vi "Process.vi"(0 "reference in":refnum<class "Script.lvclass">, 5 "error in":errorcluster) -> (14 "reference out":refnum<class "Script.lvclass">, 19 "error out":errorcluster)   [LabVIEW 2023, in "Script.lvclass"]
uses:
  Script.lvclass
  Script.lvclass/Script.ctl
  <vilib>/Utility/SystemLogging/NI_SystemLogging.lvlib
panel:
  out "error info":errorcluster
  out "Last Command":string
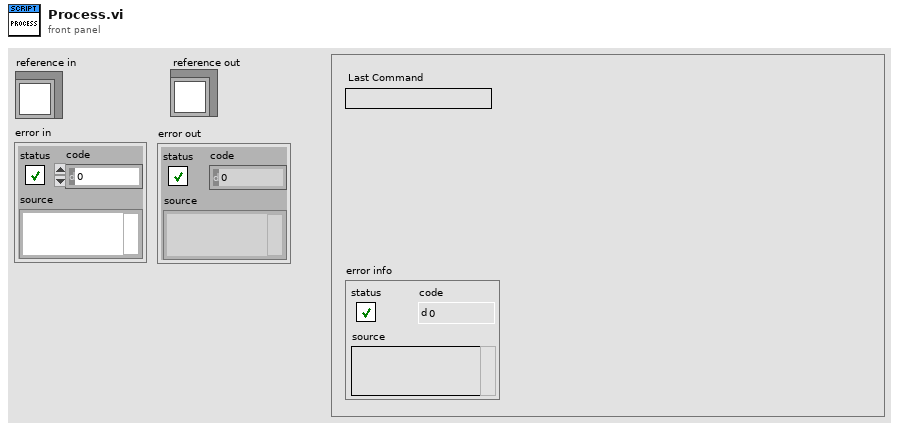
[diagram p1: front panel]
types:
  T1 = cluster{"Core":cluster{"Timeout":i32, "Events":cluster{"EventsToProcess":refnum<event-registration>}, "EventFromProcess":refnum<user-event>, "ProcessSyncQueue":refnum<queue>, "QueueFromProcess":refnum<queue>, "Command":string, "Data":variant}, "Process ID":i32, "Script Prefix":string, "Log File":string, "Full Command":string, "Script Name":string, "Console Listbox":refnum<vi>}
  T2 = enum32{"Invalid", "Standard", "Closed", "Hidden", "Minimized", "Maximized"}
  T3 = cluster{"EventsToProcess":refnum<event-registration>}
  T4 = typedef "Script.lvclass/ObjectAttributes.ctl" = cluster{"Update Rate (ms)":i32, "Console Listbox":refnum<vi>, "Full Command":string, "Script Name":string, "Log File":string, "IP Address":string}
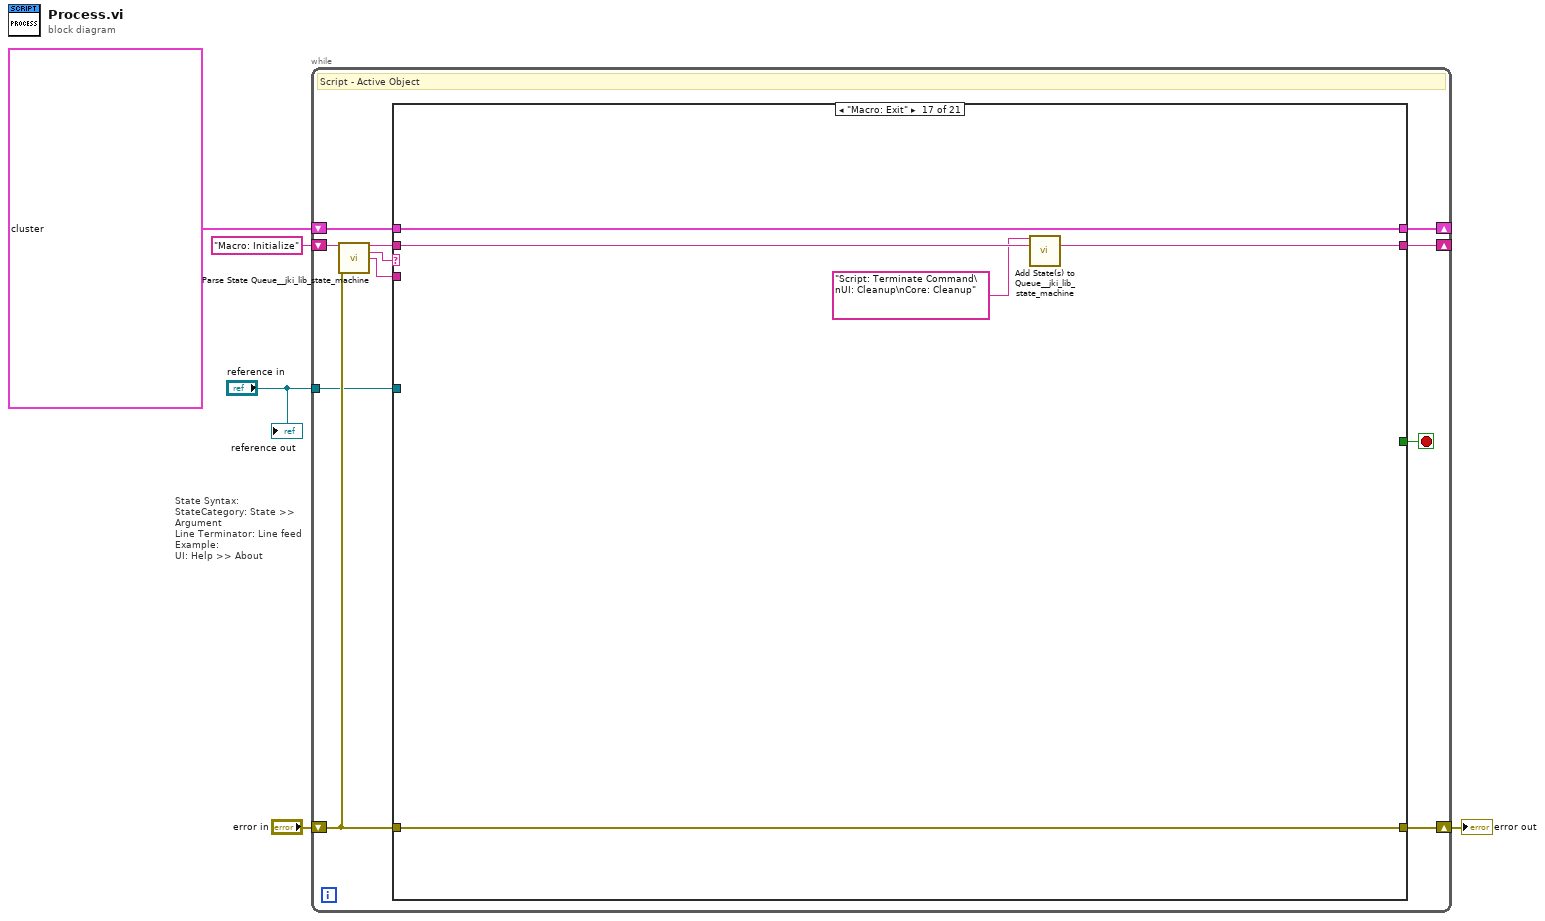
[diagram p0: block diagram]
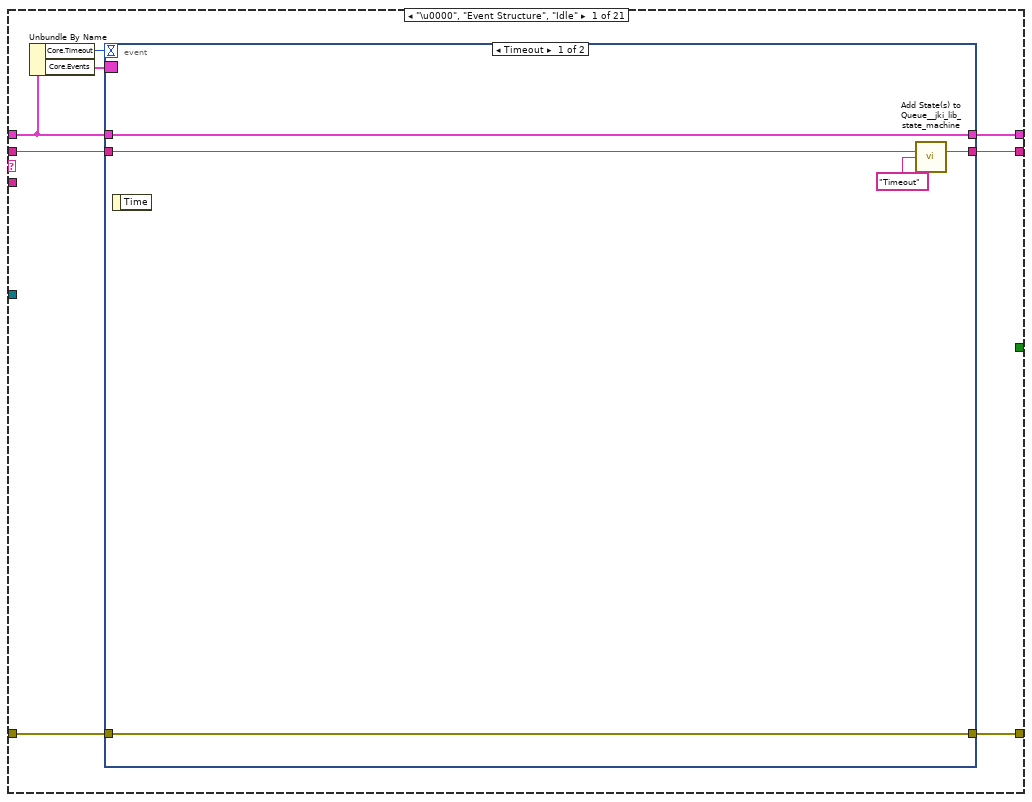
[diagram p2: hidden frame]
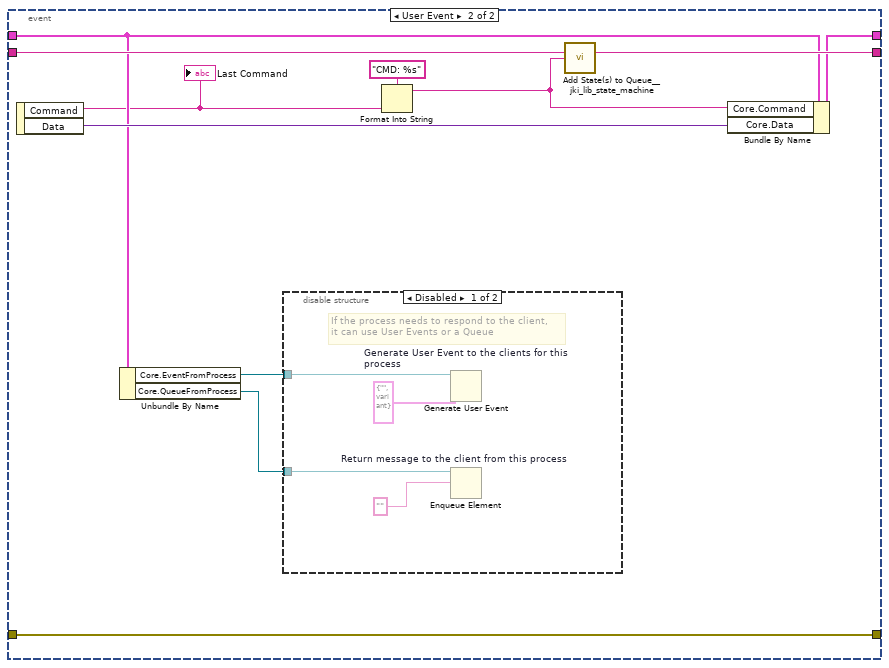
[diagram p3: hidden frame]
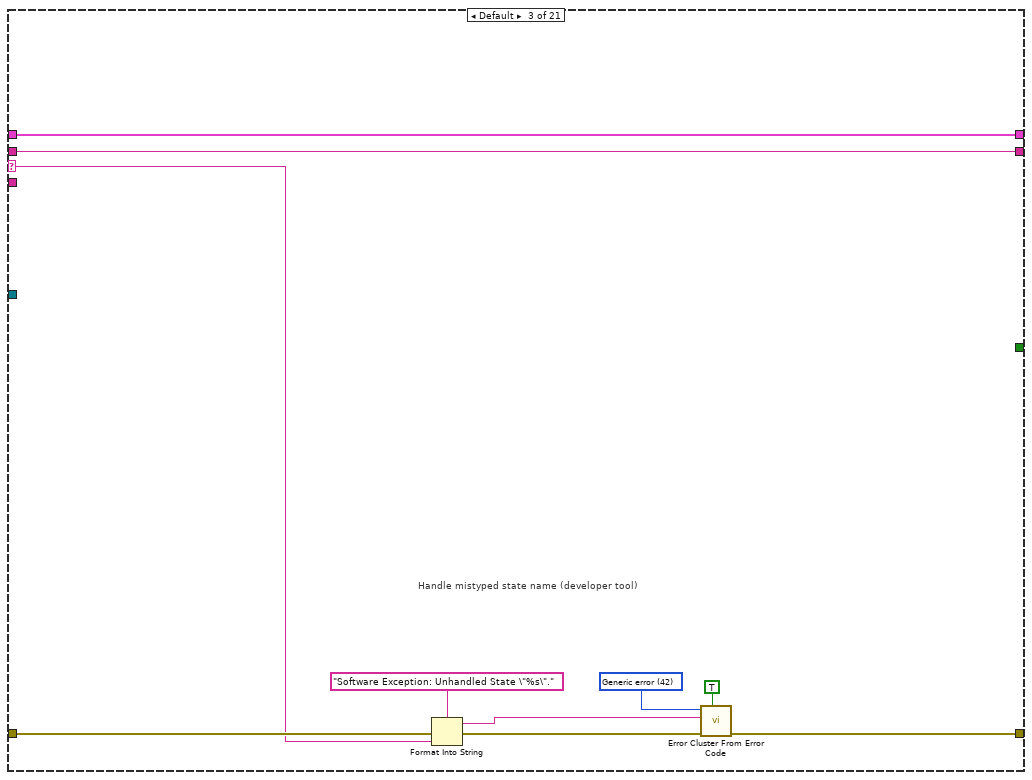
[diagram p6: hidden frame]
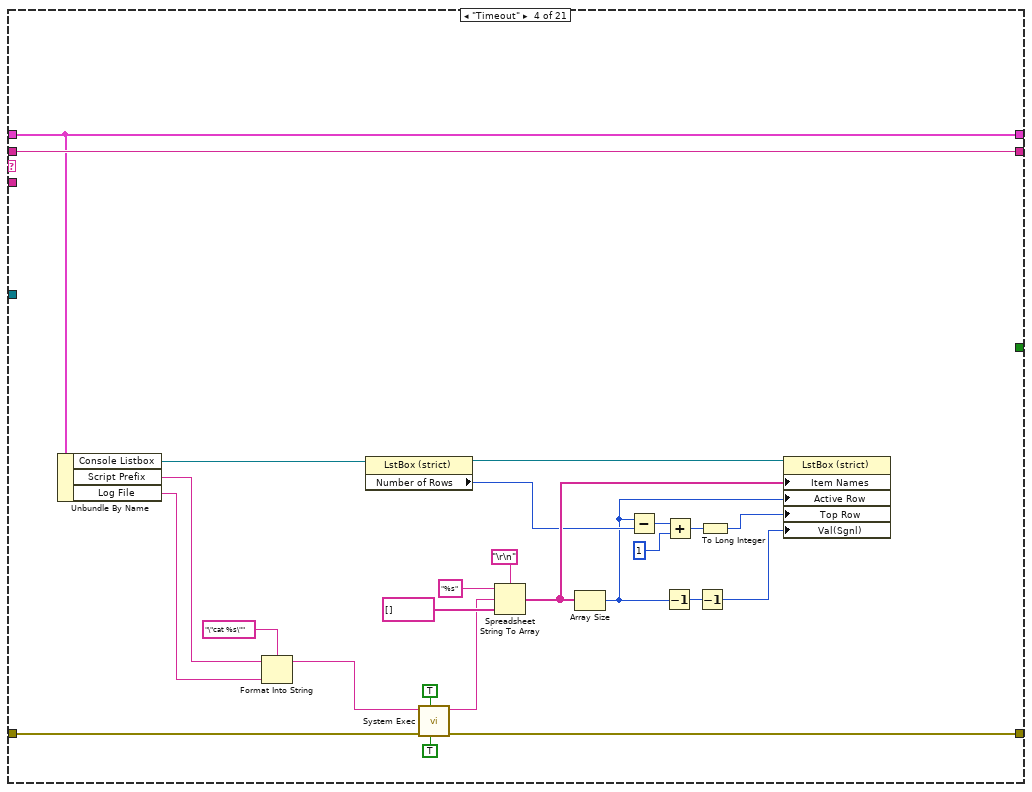
[diagram p7: hidden frame]
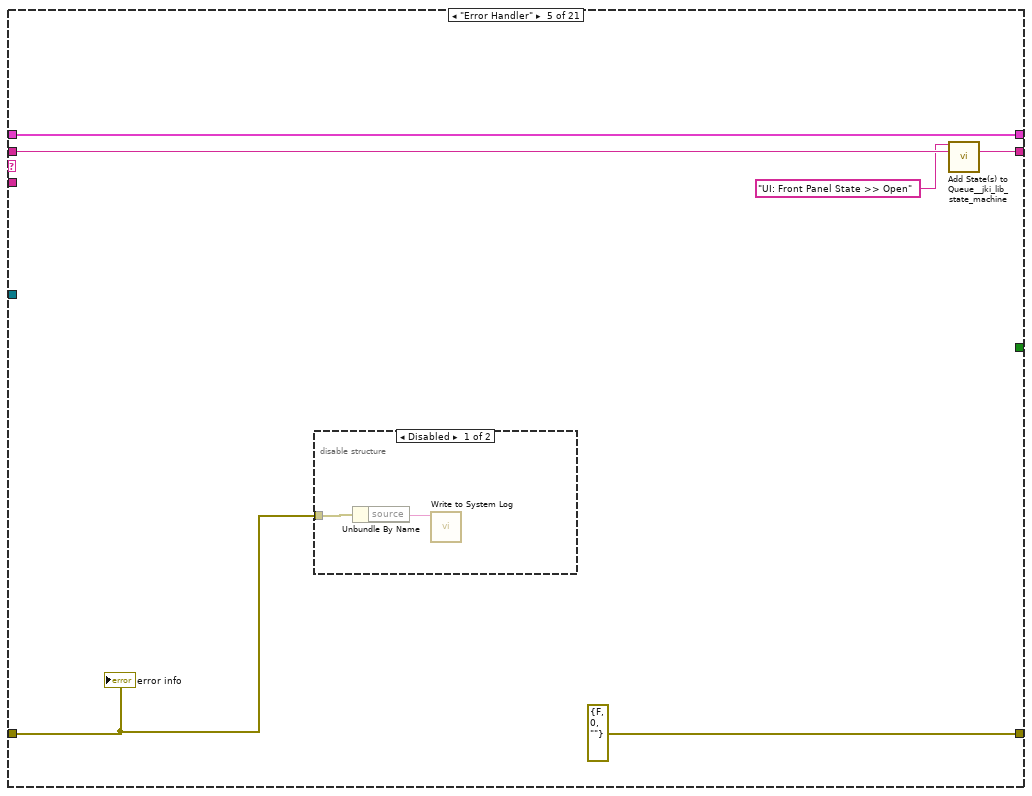
[diagram p8: hidden frame]
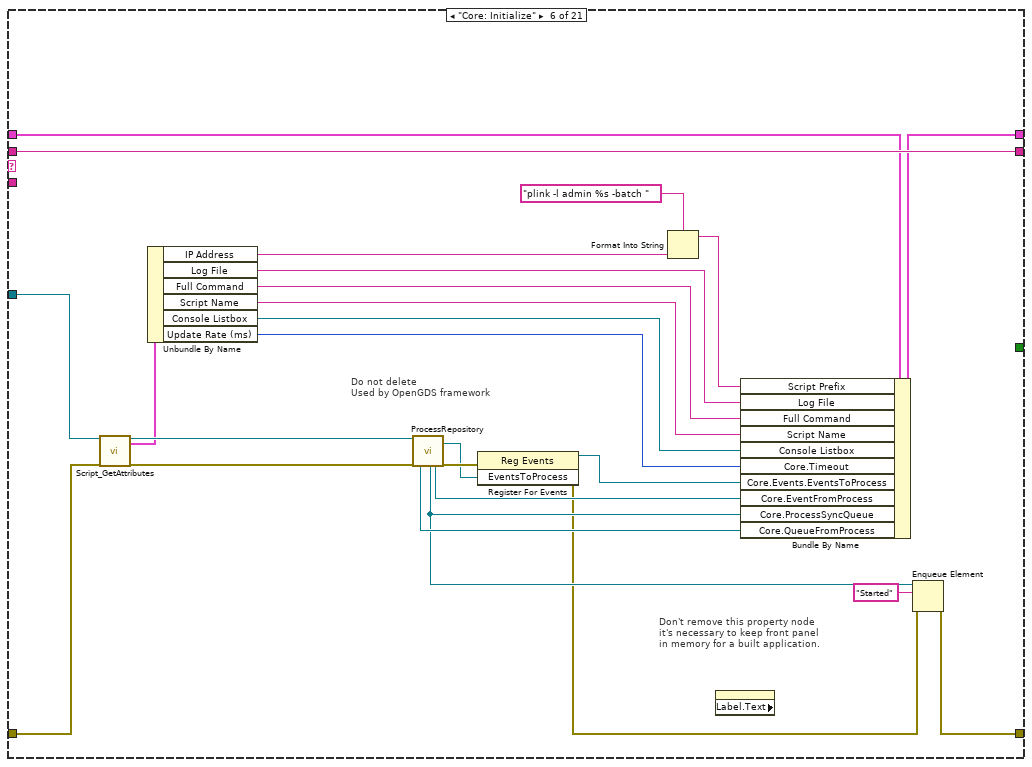
[diagram p10: hidden frame]
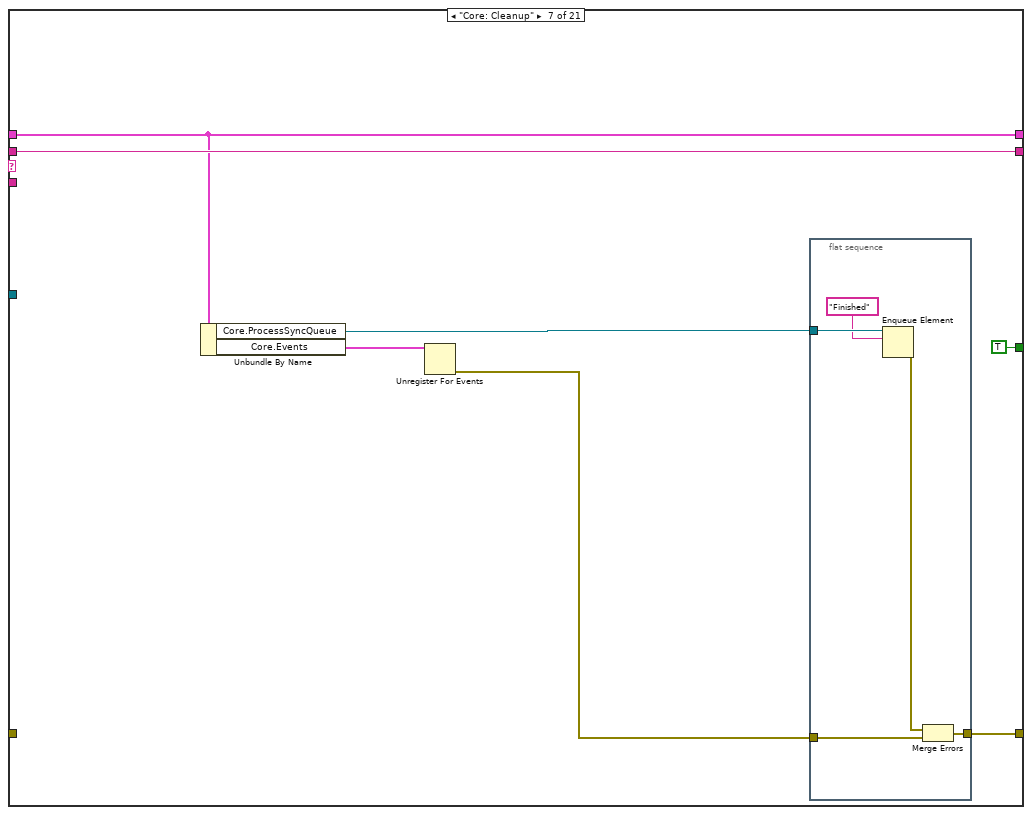
[diagram p11: hidden frame]
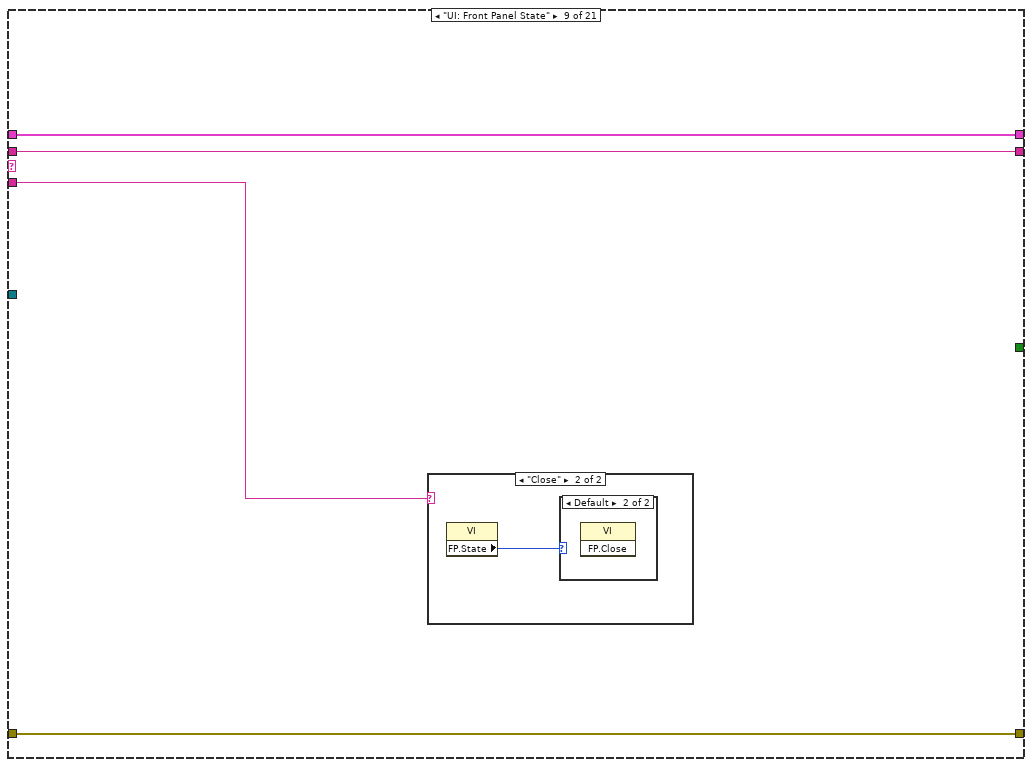
[diagram p13: hidden frame]
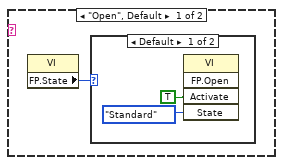
[diagram p14: hidden frame]
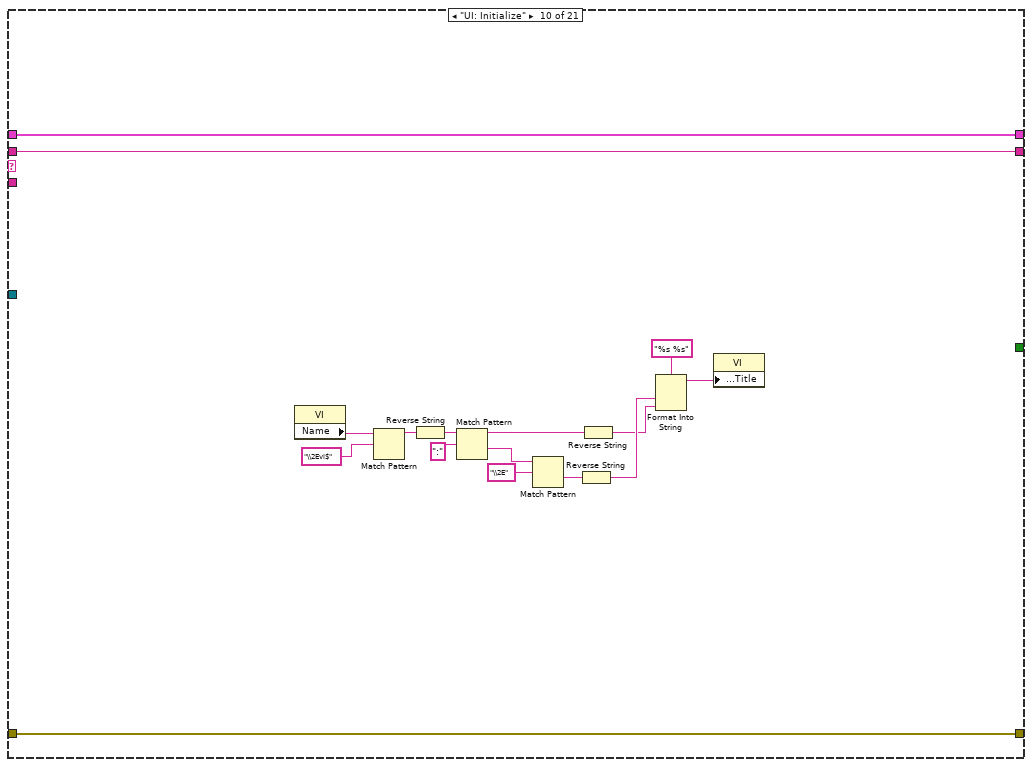
[diagram p17: hidden frame]
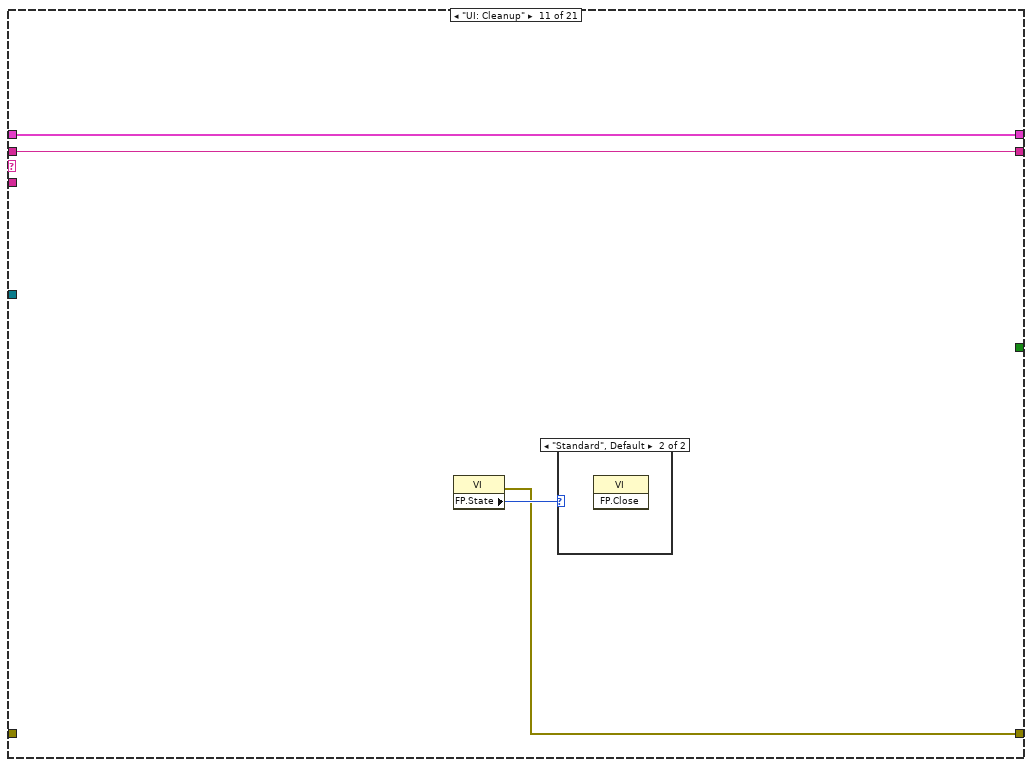
[diagram p18: hidden frame]
diagram:
  # "State Syntax:\nStateCategory: State >> Argument\nLine Terminator: Line feed\nExample:\nUI: Help >> About"
  n1 = while {
    shift-right: [w15] -> w4
    shift-left: "error in" -> [w16]
    shift-right: [w8] -> _
    shift-left: "Macro: Initialize" ("States Out") -> [w11]
    shift-right: [w14] -> _
    shift-left: T1 {"Core"={"Timeout"=-1, "Events"={"EventsToProcess"=refnum}, "EventFromProcess"=refnum, "ProcessSyncQueue"=refnum, "QueueFromProcess"=refnum, "Command"="", "Data"=variant}, "Process ID"=0, "Script Prefix"="", "Log File"="", "Full Command"="", "Script Name"="", "Console Listbox"=refnum} ("LocalVariables") -> [w13]
    tunnel: "reference in" -> [w6]
    stop <- w7 stop-if-true
    # "Script - Active Object"
    n2 = call <vilib>:"Parse State Queue__jki_lib_state_machine.vi"("State Queue"=w11, "Error In (no error)"=w16) -> ("Remaining States"=w10:string, "Current State"=w12:string, "Arguments"=w9:string)  [unwired: 11 in]
    n3 = case shown="\"Macro: Exit\"" w12 {
      selector: w12 -> [_ _ w48 _ _ _ _ _ _ _ _ _ _ _ _ _ _ _ _ _ _]
      tunnel: w16 -> [w18 w47 w50 w63 w84 w101 _ w130 w131 w154 _ w161 w164 w171 w172 w178 w183 w185 w193 w202 w219]
      tunnel: [w19 w47 w49 w62 errorcluster {"status"=FALSE, "code"=0, "source"=""} ("error constant") w115 w118 w130 w131 w154 w155 w161 w164 w171 w172 w178 w183 w185 w192 w201 w217] -> w15
      tunnel: [w24 w46 w57 w61 w88 w113 w119 w129 w133 w146 w156 w160 w163 w170 w173 w179 w184 w186 w190 w203 w216] -> w14
      tunnel: w13 -> [w20 w46 w57 w61 w88 w112 w119 w129 w133 w146 w156 w160 w163 w170 w173 w179 w184 w186 w191 w203 w216]
      tunnel: w10 -> [w22 w45 w56 w82 w87 w114 w122 w128 w134 w153 w158 w159 _ w169 w174 w177 w182 w187 w200 w209 w221]
      tunnel: w9 -> [_ _ _ _ _ _ _ _ w132 _ _ _ _ w166 _ _ _ _ _ _ _]
      tunnel: [w21 w45 w56 w82 w86 w114 w122 w128 w134 w153 w158 w159 "Macro: Exit" ("State(s) at Back (\"\")") w168 w174 w176 w181 w187 w200 w209 w221] -> w8
      tunnel: [_ _ _ _ _ _ TRUE _ _ _ _ _ _ _ _ _ _ _ _ _ _] -> w7
      tunnel: w6 -> [_ _ _ _ _ w103 _ _ _ _ _ _ _ _ _ _ _ _ _ _ _]
      frame "\u0000", "Event Structure", "Idle" {
        n4 = Unbundle By Name(w20) -> ("Core.Timeout"=w17:i32, "Core.Events"=w23:T3)
        n5 = event shown="[0] Timeout" {
          selector: w23 -> [_ _]
          dyn-events: _ -> [_ _]
          timeout: w17 -> [_ _]
          tunnel: w20 -> [w29 w33]
          tunnel: [w29 w38] -> w24
          tunnel: [w27 w40] -> w21
          tunnel: w22 -> [w28 w39]
          tunnel: [w25 w34] -> w19
          tunnel: w18 -> [w25 w34]
          event Timeout {
            n6 = event-data() -> ()  [unwired: 1 in, 1 out]
            n7 = call <vilib>:"Add State(s) to Queue__jki_lib_state_machine.vi"("State(s) in (\"\")"=w28, "State(s) at Back (\"\")"="Timeout" ("State(s) at Back (\"\")")) -> ("States Out"=w27:string)  [unwired: 13 in]
          }
          event User Event {
            n8 = event-data() -> ("Command"=w31:string, "Data"=w37:variant)  [unwired: 1 in]
            "Last Command" <- w31
            n9 = Unbundle By Name(w33) -> ("Core.EventFromProcess"=w36:refnum<user-event>, "Core.QueueFromProcess"=w35:refnum<queue>)
            n10 = disable-structure shown="Disabled" {
              disable-tunnel: w36 -> [w44 _]
              disable-tunnel: w35 -> [w43 _]
              frame Disabled {
                # "If the process needs to respond to the client,\nit can use User Events or a Queue"
                n11 = Generate User Event "Generate User Event to the clients for this process"(user event=w44, event data cluster=cluster{"Command":string, "Data":variant} {"Command"="", "Data"=variant} ("event data")) -> ()  [unwired: 2 in, 2 out]
                n12 = Enqueue Element "Return message to the client from this process"(queue=w43, element="") -> ()  [unwired: 2 in, 3 out]
              }
              frame Enabled {
              }
            }
            n13 = Format Into String(format string="CMD: %s", w31) -> (resulting string=w30:string)  [unwired: 2 in, 1 out]
            n14 = call <vilib>:"Add State(s) to Queue__jki_lib_state_machine.vi"("State(s) in (\"\")"=w39, "State(s) at Back (\"\")"=w30) -> ("States Out"=w40:string)  [unwired: 13 in]
            n15 = Bundle By Name(cluster=w33, "Core.Command"=w30, "Core.Data"=w37) -> (w38:T1)
          }
        }
      }
      frame "---------- Core ----------" {
      }
      frame Default {
        w54 = 42 items=["No error", "Argument error", "Memory is full", "Out of zone", "End of file", "File already open", "Generic file I/O error", "File not found", "File permission error", "Disk is full", "Duplicate path", "Too many files open", "System feature not enabled", "Resource file not found", "Cannot add resource", "Resource not found", "Image not found", "Image memory error", "Pen does not exist", "Config type invalid", "Config token not found", "Config parse error", "Config memory error", "Bad external code format", "Bad external code offset", "External code not present", "Null window", "Destroy window error", "Null menu", "Print aborted", "Bad print record", "Print driver error", "Windows error during printing", "Memory error during printing", "Print dialog error", "Generic print error", "Invalid device refnum", "Device not found", "Device parameter error", "Device unit error", "Cannot open device", "Device call aborted", "Generic error", "Cancelled by user", "Object ID too low", "Object ID too high", "Object not in heap", "Unknown heap", "Unknown object (invalid DefProc)", "Unknown object (DefProc not in table)", "Message out of range", "Invalid (null) method", "Unknown message", "Manager call not supported", "Bad address", "Network operation in progress", "Network operation timed out", "Connection is busy", "Network attribute not supported", "Network error", "Address in use", "System out of memory", "Connection aborted", "Connection refused", "Not connected", "Already connected", "Connection closed", "Initialization error (interapplication manager)", "Bad occurrence", "Wait on unbound occurrence handler", "Occurrence queue overflow", "Datalog type conflict", "Unused", "Unrecognized type (interapplication manager)", "Memory corrupt", "Failed to make temporary DLL", "Old CIN version", "Drag socket not found", "Failed to load drop-object", "Failed to register OLE object", "Failed to release OLE object", "Format specifier type mismatch", "Unknown format specifier", "Too few format specifiers", "Too many format specifiers", "Scan failed", "Newer CIN version", "Error converting to variant", "Runtime menu error", "Password tampered", "Variant attribute not found", "Incompatible variant data type", "Event data is not available", "Event Store is not present", "Occurrence is not found", "Event Queue is not created", "Event info is not available", "Refnum passed is NULL", "Error retrieving Class GUID", "Error retrieving CoClass GUID", "Error retrieving TypeLib GUID.", "Bad built application magic bytes.", "Specific driver is different from the specific driver associated with the Logical Name.", "There is no session opened to the class driver.", "Max Error", "MAX - Error with config objects", "MAX - Error loading configuration", "MAX - Group not supported"]
        # "Handle mistyped state name (developer tool)"
        n16 = Format Into String(format string="Software Exception: Unhandled State \"%s\"." ("message"), error in=w50, w48) -> (resulting string=w53:string, error out=w52:errorcluster)  [unwired: 1 in]
        n17 = call <vilib>:"Error Cluster From Error Code.vi"("show call chain? (False)"=TRUE, "error in (no error)"=w52, "error message (\"\")"=w53, "error code (0)"=w54) -> ("error out"=w49:errorcluster)  [unwired: 5 in]
      }
      frame "Timeout" {
        n18 = Unbundle By Name(w61) -> ("Console Listbox"=w60:refnum<vi>, "Script Prefix"=w58:string, "Log File"=w59:string)
        n19 = Format Into String(format string="\"cat %s\"", initial string=w58, w59) -> (resulting string=w78:string)  [unwired: 1 in, 1 out]
        n20 = property class="LstBox (strict)"(reference=w60) -> (reference out=w73:refnum<vi>, "Number of Rows"=w67:u32)  [unwired: 1 in, 1 out]
        n21 = call <vilib>:"System Exec.vi"("run minimized? (F)"=TRUE, "wait until completion? (T)"=TRUE, "error in (no error)"=w63, "command line"=w78) -> ("error out"=w62:errorcluster, "standard output"=w76:string)  [unwired: 4 in, 2 out]
        n22 = Spreadsheet String To Array(delimiter (Tab)="\r\n", format string="%s", spreadsheet string=w76, array type (2D Dbl)=string[] []) -> (array=w68:string[])
        n23 = Array Size(array=w68) -> (size(s)=w65:i32)
        n24 = Subtract(x=w65, y=w67) -> (x-y=w72:u32)
        n25 = Decrement(x=w65) -> (x-1=w64:i32)
        n26 = Add(x=w72, y=u32 1) -> (x+y=w70:u32)
        n27 = Decrement(x=w64) -> (x-1=w66:i32)
        n28 = To Long Integer(number=w70) -> (32bit integer=w69:i32)
        n29 = property class="LstBox (strict)"(reference=w73, "Item Names"=w68, "Active Row"=w65, "Top Row"=w69, "Val(Sgnl)"=w66) -> ()  [unwired: 1 in, 2 out]
      }
      frame "Error Handler" {
        n30 = disable-structure shown="Disabled" {
          disable-tunnel: w84 -> [w90 _]
          frame Disabled {
            n31 = Unbundle By Name(w90) -> ("source"=w89:string)
            n32 = call <vilib>:"Write to System Log.vi"("message"=w89) -> ()  [unwired: 10 in, 1 out]
          }
          frame Enabled {
          }
        }
        n33 = call <vilib>:"Add State(s) to Queue__jki_lib_state_machine.vi"("State(s) in Front (\"\")"="UI: Front Panel State >> Open" ("State(s) at Back (\"\")"), "State(s) in (\"\")"=w87) -> ("States Out"=w86:string)  [unwired: 13 in]
        "error info" <- w84
      }
      frame "Core: Initialize" {
        # "Do not delete\nUsed by OpenGDS framework"
        # "Don't remove this property node\nit's necessary to keep front panel\nin memory for a built application."
        # "Template created by VI Technologies"
        n34 = call "Script_GetAttributes.vi"("reference in"=w103, "Error In"=w101) -> ("reference out"=w102:refnum<class "Script.lvclass">, "Data"=w97:T4, "Error Out"=w100:errorcluster)  [unwired: 14 in, 1 out]
        n35 = Unbundle By Name(w97) -> ("IP Address"=w96:string, "Log File"=w95:string, "Full Command"=w94:string, "Script Name"=w93:string, "Console Listbox"=w91:refnum<vi>, "Update Rate (ms)"=w92:i32)
        n36 = call "ProcessRepository.vi"("reference in"=w102, "Error In"=w100) -> ("QueueFromProcess"=w107:refnum<queue>, "ProcessSyncQueue"=w105:refnum<queue>, "EventFromProcess"=w108:refnum<user-event>, "EventsToProcess"=w110:refnum<user-event>, "Error Out"=w111:errorcluster)  [unwired: 10 in, 3 out]
        n37 = register-events(error in=w111, w110) -> (reference out=w109:refnum<event-registration>, error out=w104:errorcluster)  [unwired: 1 in]
        n38 = Format Into String(format string="plink -l admin %s -batch ", w96) -> (resulting string=w98:string)  [unwired: 2 in, 1 out]
        n39 = property on="reference in" class="LVClassControl (strict)" props=["Label", "Text"]() -> ()  [unwired: 2 in, 3 out]
        n40 = Bundle By Name(cluster=w112, "Script Prefix"=w98, "Log File"=w95, "Full Command"=w94, "Script Name"=w93, "Console Listbox"=w91, "Core.Timeout"=w92, "Core.Events.EventsToProcess"=w109, "Core.EventFromProcess"=w108, "Core.ProcessSyncQueue"=w105, "Core.QueueFromProcess"=w107) -> (w113:T1)
        n41 = Enqueue Element(queue=w105, element="Started", error in (no error)=w104) -> (error out=w115:errorcluster)  [unwired: 1 in, 2 out]
      }
      frame "Core: Cleanup" {
        n42 = Unbundle By Name(w119) -> ("Core.ProcessSyncQueue"=w120:refnum<queue>, "Core.Events"=w117:T3)
        n43 = Unregister For Events(event registration refnum=w117) -> (error out=w116:errorcluster)  [unwired: 1 in]
        n44 = flat-sequence {
          tunnel: [w126] -> w118
          tunnel: w120 -> [w125]
          tunnel: w116 -> [w124]
          frame #0 {
            n45 = Enqueue Element(queue=w125, element="Finished") -> (error out=w127:errorcluster)  [unwired: 2 in, 2 out]
            n46 = Merge Errors(w127, w124) -> (w126:errorcluster)
          }
        }
      }
      frame "---------- UI ----------" {
      }
      frame "UI: Front Panel State" {
        n47 = case shown="\"Close\"" w132 {
          frame "Open", Default {
            n48 = property class="VI"() -> ("FP.State"=w135:T2)  [unwired: 2 in, 2 out]
            n49 = case shown="Default" w135 {
              frame Default {
                n50 = invoke class="VI" method="FP.Open"("Activate"=TRUE, "State"=T2."Standard") -> ()  [unwired: 3 in, 5 out]
              }
              frame "Standard" {
              }
            }
          }
          frame "Close" {
            n51 = property class="VI"() -> ("FP.State"=w138:T2)  [unwired: 2 in, 2 out]
            n52 = case shown="Default" w138 {
              frame "Closed" {
              }
              frame Default {
                n53 = invoke class="VI" method="FP.Close"() -> ()  [unwired: 3 in, 3 out]
              }
            }
          }
        }
      }
      frame "UI: Initialize" {
        n54 = property class="VI"() -> ("Name"=w152:string)  [unwired: 2 in, 2 out]
        n55 = Match Pattern(string=w152, regular expression="\\2Evi$") -> (before substring=w150:string)  [unwired: 1 in, 3 out]
        n56 = Reverse String(1:w150) -> (0:w149:string)
        n57 = Match Pattern(string=w149, regular expression=":") -> (before substring=w147:string, after substring=w145:string)  [unwired: 1 in, 2 out]
        n58 = Match Pattern(string=w145, regular expression="\\2E") -> (after substring=w143:string)  [unwired: 1 in, 3 out]
        n59 = Reverse String(1:w143) -> (0:w142:string)
        n60 = Reverse String(1:w147) -> (0:w141:string)
        n61 = Format Into String(format string="%s %s", w142, w141) -> (resulting string=w140:string)  [unwired: 2 in, 1 out]
        n62 = property class="VI"("Front Panel.Title"=w140) -> ()  [unwired: 2 in, 2 out]
      }
      frame "UI: Cleanup" {
        n63 = property class="VI"() -> (error out=w155:errorcluster, "FP.State"=w157:T2)  [unwired: 2 in, 1 out]
        n64 = case shown="\"Standard\", Default" w157 {
          frame "Closed" {
          }
          frame "Standard", Default {
            n65 = invoke class="VI" method="FP.Close"() -> ()  [unwired: 3 in, 3 out]
          }
        }
      }
      frame "---------- CMD ----------" {
      }
      frame "CMD: Exit" {
      }
      frame "CMD: Front Panel State" {
        n66 = Format Into String(format string="UI: Front Panel State>>%s" ("string"), w166) -> (resulting string=w165:string)  [unwired: 2 in, 1 out]
        n67 = call <vilib>:"Add State(s) to Queue__jki_lib_state_machine.vi"("State(s) in (\"\")"=w169, "State(s) at Back (\"\")"=w165) -> ("States Out"=w168:string)  [unwired: 13 in]
      }
      frame "---------- Macro ----------" {
      }
      frame "Macro: Initialize" {
        n68 = call <vilib>:"Add State(s) to Queue__jki_lib_state_machine.vi"("State(s) in Front (\"\")"="Core: Initialize\nUI: Initialize\nScript: Check Running\nScript: Run Command\nScript: Check Running" ("States Out"), "State(s) in (\"\")"=w177) -> ("States Out"=w176:string)  [unwired: 13 in]
      }
      frame "Macro: Exit" {
        n69 = call <vilib>:"Add State(s) to Queue__jki_lib_state_machine.vi"("State(s) in Front (\"\")"="Script: Terminate Command\nUI: Cleanup\nCore: Cleanup", "State(s) in (\"\")"=w182) -> ("States Out"=w181:string)  [unwired: 13 in]
      }
      frame "---------- Script ----------" {
      }
      frame "Script: Check Running" {
        n70 = Unbundle By Name(w191) -> ("Script Prefix"=w188:string, "Script Name"=w189:string)
        n71 = Format Into String(format string="\"pgrep %s\"", initial string=w188, w189) -> (resulting string=w196:string)  [unwired: 1 in, 1 out]
        n72 = call <vilib>:"System Exec.vi"("run minimized? (F)"=TRUE, "wait until completion? (T)"=TRUE, "error in (no error)"=w193, "command line"=w196) -> ("error out"=w192:errorcluster, "standard output"=w195:string)  [unwired: 4 in, 2 out]
        n73 = Decimal String To Number(string=w195) -> (number=w194:i32)  [unwired: 2 in, 1 out]
        n74 = Bundle By Name(cluster=w191, "Process ID"=w194) -> (w190:T1)
      }
      frame "Script: Run Command" {
        n75 = Unbundle By Name(w203) -> ("Process ID"=w208:i32, "Script Prefix"=w204:string, "Full Command"=w205:string)
        n76 = Format Into String(format string="\"%s\"", initial string=w204, w205) -> (resulting string=w206:string)  [unwired: 1 in, 1 out]
        n77 = case shown="0" w208 {
          tunnel: w202 -> [w210 w213]
          tunnel: [w210 w212] -> w201
          tunnel: w206 -> [_ w211]
          frame Default {
            # "process already running\ndont launch again"
          }
          frame 0 {
            # "process not running\nlaunch it"
            n78 = call <vilib>:"System Exec.vi"("run minimized? (F)"=TRUE, "wait until completion? (T)"=FALSE, "error in (no error)"=w213, "command line"=w211) -> ("error out"=w212:errorcluster)  [unwired: 4 in, 3 out]
          }
        }
      }
      frame "Script: Terminate Command" {
        n79 = Unbundle By Name(w216) -> ("Script Prefix"=w218:string, "Process ID"=w220:i32)
        n80 = case shown="Default" w220 {
          selector: w220 -> [w224 _]
          tunnel: w219 -> [w227 w230]
          tunnel: [w226 w230] -> w217
          tunnel: w218 -> [w222 _]
          frame Default {
            n81 = Format Into String(format string="\"kill %d\"", initial string=w222, w224) -> (resulting string=w223:string)  [unwired: 1 in, 1 out]
            n82 = call <vilib>:"System Exec.vi"("run minimized? (F)"=TRUE, "wait until completion? (T)"=TRUE, "error in (no error)"=w227, "command line"=w223) -> ("error out"=w226:errorcluster)  [unwired: 4 in, 3 out]
          }
          frame 0 {
            # "process not running\nnothing to terminate"
          }
        }
      }
    }
  }
  "error out" <- w4
  "reference out" <- "reference in"
